vi "IR_Data_Save.vi"(8 "error in (no error)":errorcluster caption="错误输入（无错误）", 10 "AC_SET DATA":string[](array[string])) -> (0 "error out":errorcluster caption="错误输出", 2 "布尔":bool, 3 "out string":string)   [LabVIEW 2018]
panel:
  in  "FALL TIME:":string
  in  "停止":bool
  in  "按钮":bool
  in  "REMP TIME:":string
  in  "FALL TIME:":string
  in  "TEST TIME:":string
  in  "LOW LIMT:":string
  in  "HIGH LIMT:":string
  in  "VIKTAGE:":string
  # "IR参数设置"
  # "mA(0.001~10mA)"
  # "mA(0~10mA)"
  # "KV(0.005~5KV)"
  # "Mohm(0.1~50Gohm)"
  # "Mohm(0.1~50Gohm)"
  # "S(0.1~999S)"
  # "S(0.3~999S)"
  # "S(0.1~999S)"
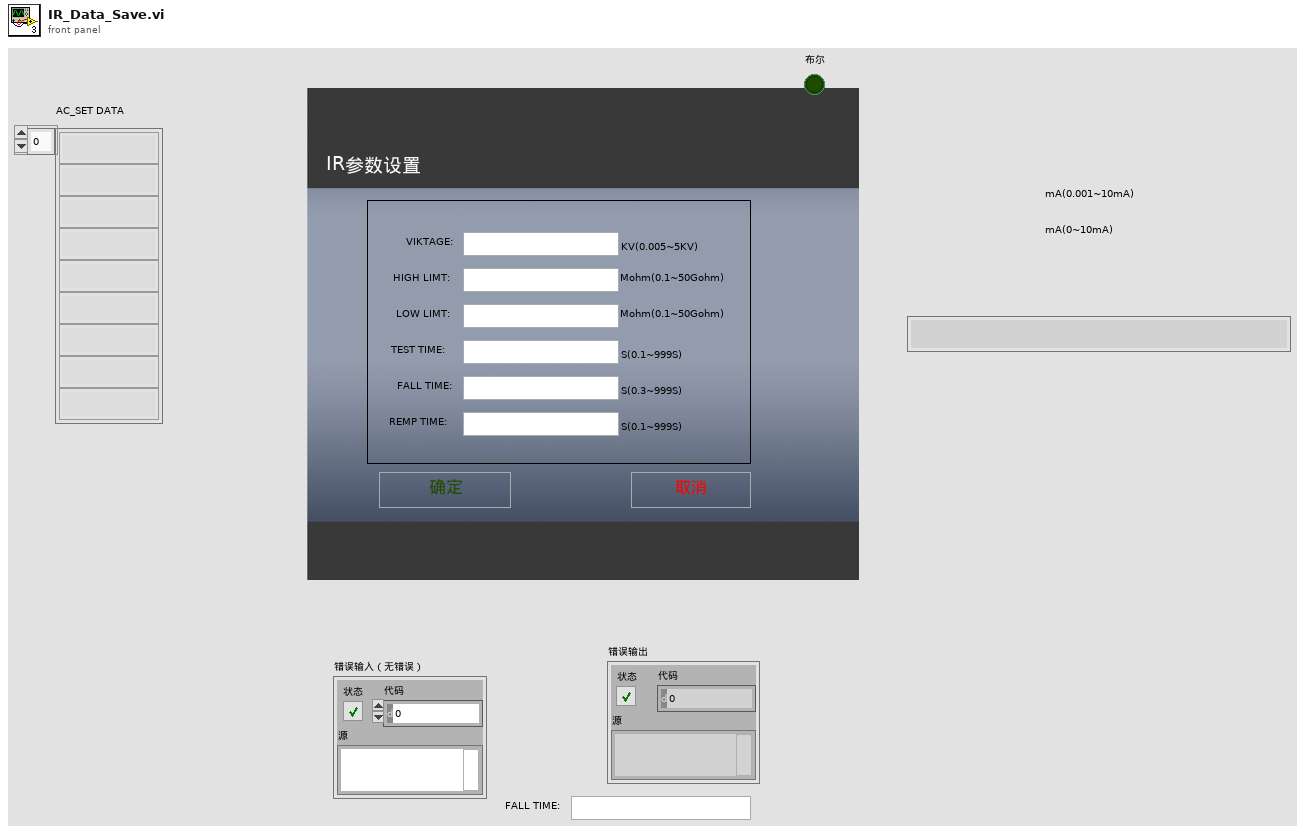
[diagram p1: front panel]
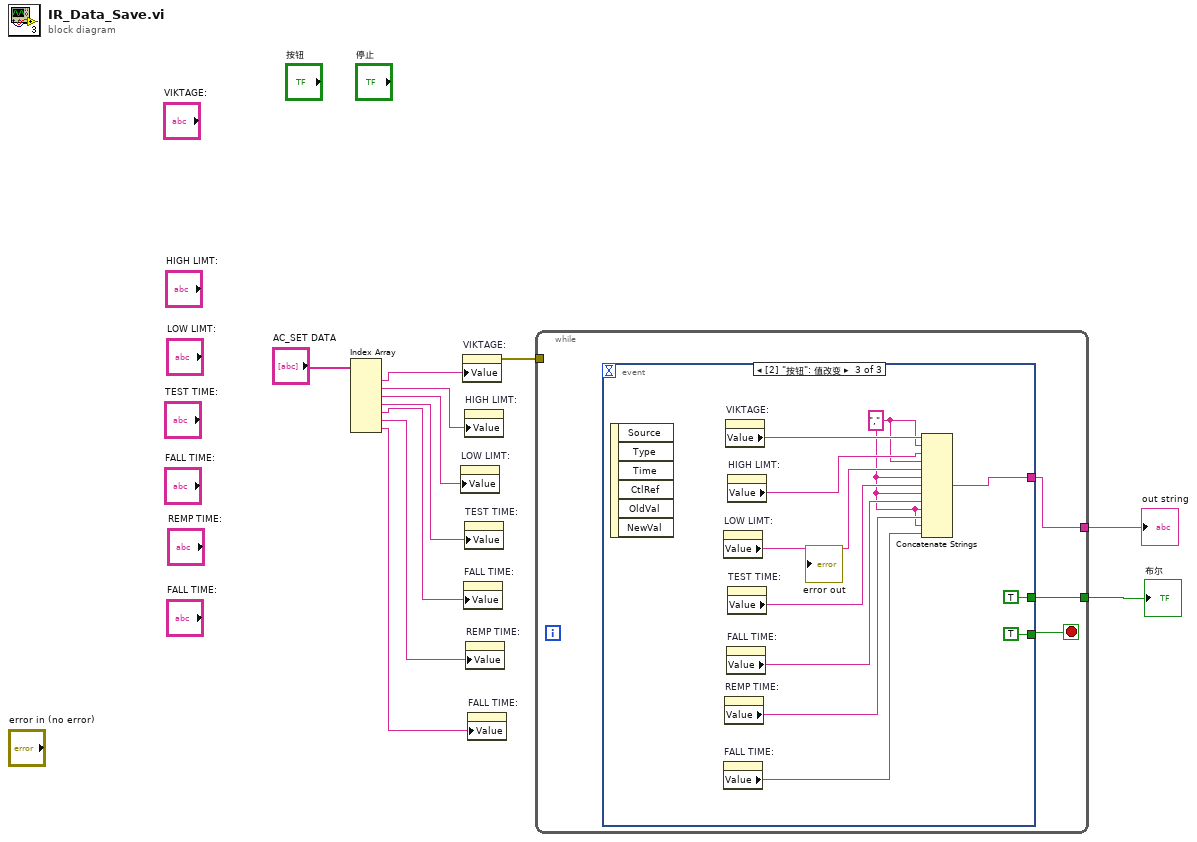
[diagram p0: block diagram]
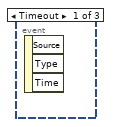
[diagram p2: hidden frame]
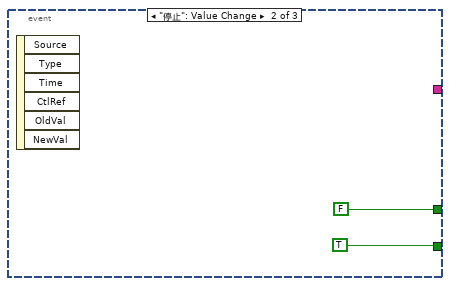
[diagram p3: hidden frame]
diagram:
  n1 = Index Array(array="AC_SET DATA") -> (element #1=w10:string, element #2=w9:string, element #3=w8:string, element #4=w7:string, element #5=w6:string, element #6=w5:string, element #7=w2:string)  [unwired: 7 in]
  n2 = property on="LOW LIMT:" class="Str"("Value"=w8) -> ()  [unwired: 2 in, 2 out]
  n3 = property on="VIKTAGE:" class="Str"("Value"=w10) -> (error out=w1:errorcluster)  [unwired: 2 in, 1 out]
  n4 = property on="FALL TIME:" class="Str"("Value"=w6) -> ()  [unwired: 2 in, 2 out]
  n5 = property on="HIGH LIMT:" class="Str"("Value"=w9) -> ()  [unwired: 2 in, 2 out]
  n6 = property on="TEST TIME:" class="Str"("Value"=w7) -> ()  [unwired: 2 in, 2 out]
  n7 = property on="REMP TIME:" class="Str"("Value"=w5) -> ()  [unwired: 2 in, 2 out]
  n8 = property on="FALL TIME:" class="Str"("Value"=w2) -> ()  [unwired: 2 in, 2 out]
  n9 = while {
    tunnel: [w13] -> w4
    tunnel: [w12] -> w3
    tunnel: w1 -> [_]
    stop <- w14 stop-if-true
    n10 = event shown="[2] \"按钮\": 值改变" {
      selector: _ -> [_ _ _]
      dyn-events: _ -> [_ _ _]
      timeout: _ -> [_ _ _]
      tunnel: [_ TRUE TRUE] -> w14
      tunnel: [_ _ w21] -> w13
      tunnel: [_ FALSE TRUE] -> w12
      event Timeout {
        n11 = event-data() -> ()  [unwired: 1 in, 3 out]
      }
      event "停止": Value Change {
        n12 = event-data() -> ()  [unwired: 1 in, 6 out]
      }
      event "按钮": Value Change {
        w18 = ","
        n13 = event-data() -> ()  [unwired: 1 in, 6 out]
        n14 = property on="LOW LIMT:" class="Str"() -> ("Value"=w24:string)  [unwired: 2 in, 2 out]
        n15 = property on="FALL TIME:" class="Str"() -> ("Value"=w17:string)  [unwired: 2 in, 2 out]
        n16 = property on="REMP TIME:" class="Str"() -> ("Value"=w27:string)  [unwired: 2 in, 2 out]
        n17 = property on="VIKTAGE:" class="Str"() -> ("Value"=w22:string)  [unwired: 2 in, 2 out]
        n18 = property on="FALL TIME:" class="Str"() -> ("Value"=w26:string)  [unwired: 2 in, 2 out]
        n19 = property on="HIGH LIMT:" class="Str"() -> ("Value"=w23:string)  [unwired: 2 in, 2 out]
        n20 = property on="TEST TIME:" class="Str"() -> ("Value"=w25:string)  [unwired: 2 in, 2 out]
        n21 = Concatenate Strings(w22, w18, w23, w18, w24, w18, w25, w18, w26, w18, w27, w18, w17) -> (w21:string)
      }
    }
  }
  "out string" <- w4
  "布尔" <- w3
